vi "PSROOT_Root Project Path.vi"() -> (2 "All Path":cluster{"Tree PNG":path})   [LabVIEW 2016]
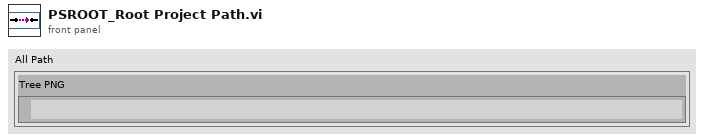
[diagram p1: front panel]
types:
  T1 = enum32{"invalid app kind", "Development System", "Run Time System", "Student Edition", "Embedded LabVIEW", "Evaluation", "Custom"}
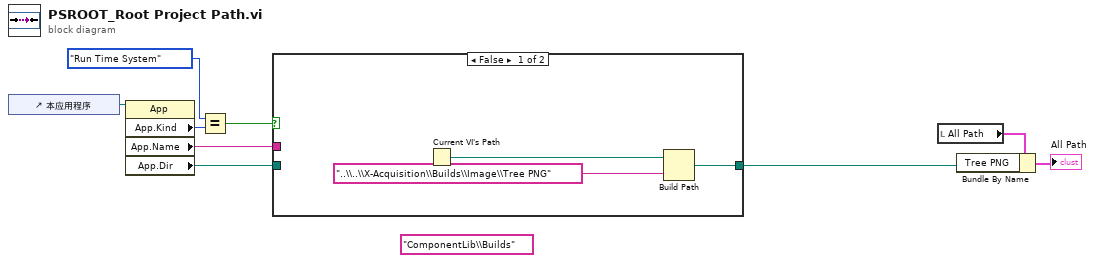
[diagram p0: block diagram]
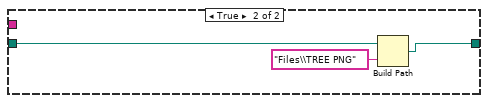
[diagram p2: hidden frame]
diagram:
  (unwired) "ComponentLib\\Builds" ("name or relative path")
  n1 = control-ref of="本应用程序"() -> (w9:refnum<vi>)
  n2 = property class="App"(reference=w9) -> ("App.Kind"=w8:T1, "App.Name"=w5:string, "App.Dir"=w4:path)  [unwired: 1 in, 2 out]
  n3 = Equal?(x=T1."Run Time System" ("应用程序:类别"), y=w8) -> (x = y?=w6:bool)
  n4 = case shown="False" w6 {
    tunnel: w5 -> [_ _]
    tunnel: w4 -> [_ w14]
    tunnel: [w11 w13] -> w1
    frame False {
      n5 = Current VI's Path() -> (path=w12:path)
      n6 = Build Path(base path=w12, name or relative path="..\\..\\X-Acquisition\\Builds\\Image\\Tree PNG") -> (appended path=w11:path)
    }
    frame True {
      n7 = Build Path(base path=w14, name or relative path="Files\\TREE PNG") -> (appended path=w13:path)
    }
  }
  n8 = local read "All Path"() -> (w3:cluster{"Tree PNG":path})
  n9 = Bundle By Name(cluster=w3, "Tree PNG"=w1) -> (→"All Path":cluster{"Tree PNG":path})
